vi "UpdateExperimentPropertiesFromTempValue.vi"(10 "temp param index":dbl, 11 "ExperimentID":string) -> ()   [LabVIEW 2017]
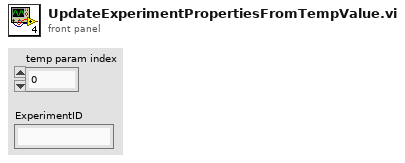
[diagram p1: front panel]
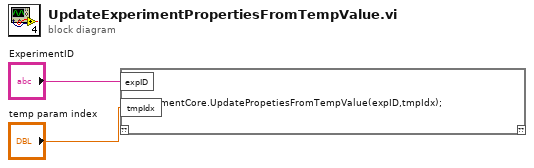
[diagram p0: block diagram]
diagram:
  n1 = script code="ExperimentCore.UpdatePropetiesFromTempValue(expID,tmpIdx);"("expID"="ExperimentID", "tmpIdx"="temp param index") -> ()  [unwired: 1 in, 1 out]
